vi "PH_Stepmotor_BaseClass.get i attribute.vi"(0 "i ref in":refnum<vi>, 5 "error in (no error)":errorcluster) -> (14 "i ref out":refnum<vi>, 16 "i attribute":T1 {"Axes PSDB Thread"."Data Status" items=["no info", "no Data collection", "no problem", "Error getting the ID", "Error writing Data", "Error getting the subsystem", "Error getting the Shot ID", "Error getting the Shot Types", "Error getting the Experiments", "Error verifying wanted Shottype", "Error verifying wanted Experiment"]}, 19 "error out":errorcluster)   [LabVIEW 2014, in "PH_Stepmotor_BaseClass.lvlib"]
doc: "Gets the i attribute data of an object.\n\nLicense Agreement for this software:\n\nCopyright (C)\nGesellschaft für Schwerionenforschung, GSI\nPlanckstr. 1\n64291 Darmstadt\nGermany\n\nContact: D.Beck@gsi.de \n\nThis program is free software; you can redistribute it and/or modify it under the terms of the GNU General Public License as published by the Free Software Foundation; either version 2 of the license, or (at your option) any later version.\n\nThis program is distributed in the hope that it will be useful, but WITHOUT ANY WARRANTY; without even the implied warranty of MERCHANTABILITY or FITNESS FOR A PARTICULAR PURPOSE. See the GNU General License for more details (http://www.gnu.org).\n\nGesellschaft für Schwerionenforschung, GSI\nPlanckstr. 1, 64291 Darmstadt, Germany\nFor all questions and ideas contact: M.Richter@gsi.de, H.Brand@gsi.de or D.Beck@gsi.de.\nLast update: 17-JUN-2004"
uses:
  PH_Stepmotor_BaseClass.lvlib
  PH_Stepmotor_BaseClass.i attribute.ctl
  PH_PSDBWriter/PH_PSDBWriter.Data Status.ctl
  PH_Stepmotor_BaseClass.Axis Attributes.ctl
  PH_Stepmotor_BaseClass.Axis Settings.ctl
  PH_Stepmotor_BaseClass.Motor Type.ctl
  PH_Stepmotor_BaseClass.Axis DIM Service IDs.ctl
  PH_Stepmotor_BaseClass.Axis Activity.ctl
  PH_Stepmotor_BaseClass.GUI Refs.ctl
  PH_PSDBWriter/PH_PSDBWriter.lvlib
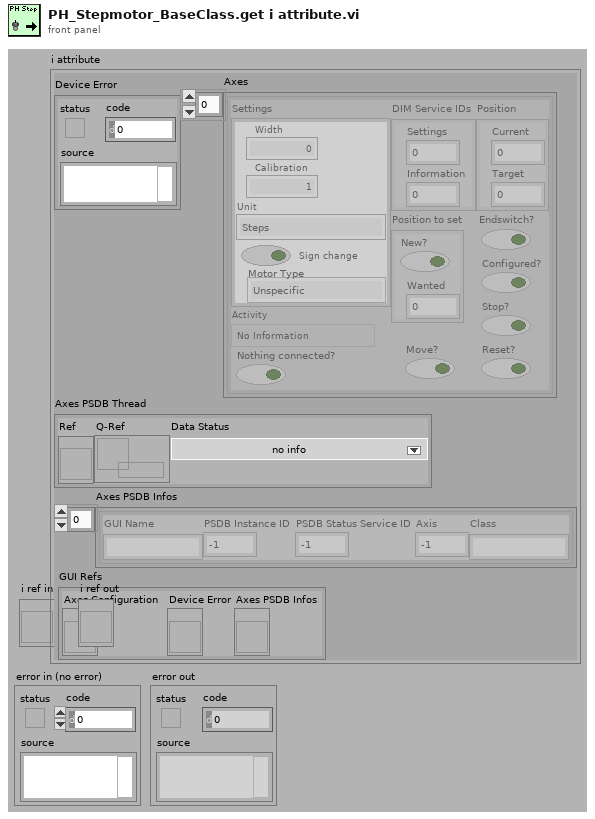
[diagram p1: front panel]
types:
  T1 = typedef "PH_Stepmotor_BaseClass.lvlib/PH_Stepmotor_BaseClass.i attribute.ctl" = cluster{"Device Error":errorcluster, "Axes PSDB Thread":cluster{"Ref":refnum<vi>, "Q-Ref":refnum<queue>, "Data Status":T2}, "Axes":T3[], "Axes PSDB Infos":cluster{"GUI Name":string, "PSDB Instance ID":i32, "PSDB Status Service ID":i32, "Axis":i32, "Class":string}[], "GUI Refs":T8}
  T2 = typedef "PH_PSDBWriter.lvlib/PH_PSDBWriter.Data Status.ctl" = i16
  T3 = typedef "PH_Stepmotor_BaseClass.lvlib/PH_Stepmotor_BaseClass.Axis Attributes.ctl" = cluster{"Settings":T4, "Endswitch?":bool, "DIM Service IDs":T6, "Activity":T7, "Configured?":bool, "Position":cluster{"Current":i32, "Target":i32}, "Position to set":cluster{"New?":bool, "Wanted":i32}, "Stop?":bool, "Reset?":bool, "Move?":bool, "Nothing connected?":bool}
  T4 = typedef "PH_Stepmotor_BaseClass.lvlib/PH_Stepmotor_BaseClass.Axis Settings.ctl" = cluster{"Sign change":bool, "Width":dbl, "Calibration":dbl, "Unit":string, "Motor Type":T5, "Unit Width":string, "Unit CF":string}
  T5 = typedef "PH_Stepmotor_BaseClass.lvlib/PH_Stepmotor_BaseClass.Motor Type.ctl" = enum16{"Unspecific", "OWIS 49.120.2633", "OWIS 49.060.1033", "OWIS 43.040.2558", "Diamond Motion 2200 series", "OWIS 49.120.266B.MV6", "Calorimeter", "Linear Stage 1", "MICOS VT-80", "MICOS VT-80 S", "Standa Rotstage nt0.95A", "PUF RA 320.200", "PUF RA 800.200", "PUF RA 800.400", "PUF RA 400.50", "1324.nn.800.50", "1324.n9c.800.50", "1324.nn.320.200", "1324.nn.400.200", "1324.nn.800.200", "1324.nn.400.50", "1324.8c9c.800.50", "1324.8c9c.400.200"}
  T6 = typedef "PH_Stepmotor_BaseClass.lvlib/PH_Stepmotor_BaseClass.Axis DIM Service IDs.ctl" = cluster{"Settings":i32, "Information":i32}
  T7 = typedef "PH_Stepmotor_BaseClass.lvlib/PH_Stepmotor_BaseClass.Axis Activity.ctl" = enum16{"No Information", "stopped", "running", "Failure", "Alarm", "stopped at backward ES", "stopped at foreward ES"}
  T8 = typedef "PH_Stepmotor_BaseClass.lvlib/PH_Stepmotor_BaseClass.GUI Refs.ctl" = cluster{"Axes Configuration":refnum<vi>, "Device Error":refnum<vi>, "Axes PSDB Infos":refnum<vi>}
  T9 = enum16{"SetAttribute", "GetAttribute", "CreateAttribute", "DestroyAttribute", "DestroyAllAtributes"}
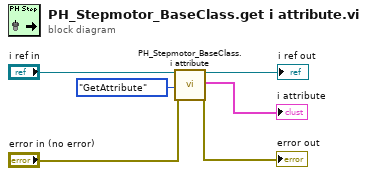
[diagram p0: block diagram]
diagram:
  n1 = call "PH_Stepmotor_BaseClass.i attribute.vi"("VI Refnum"="i ref in", "Action"=T9."GetAttribute", "error in (no error)"="error in (no error)") -> ("VI Refnum out"=→"i ref out":refnum<vi>, "CLASS.i attribute out"=→"i attribute":T1, "error out"=→"error out":errorcluster)  [unwired: 14 in]
